vi "solar_voy Pack.vi"(0 "Voyager Refnum in":T1, 1 "CMD":enum8{"CMD", "TLM"}(ring), 2 "Update Last Value? (F)":bool, 5 "TARGET":string, 7 "PACKET (\"\" = Use Variant)":string, 9 "Variant (No HDR)":variant, 11 "error in (no error)":errorcluster, 12 "Suppress Errors? (T)":bool=TRUE, 13 "HDR_GUID":string) -> (4 "Voyager Refnum out":T1, 6 "TCP Data to Send":string, 10 "Packet Index":i32, 15 "error out":errorcluster)   [LabVIEW 2018]
doc: "This packs a variant into a registered TCP packet. The variant should not include the header data. The header items are added automatically."
uses:
  <vilib>/Utility/Data Type/NI_Data Type.lvlib
  solar_voy_ctl Voyager Refnum.ctl
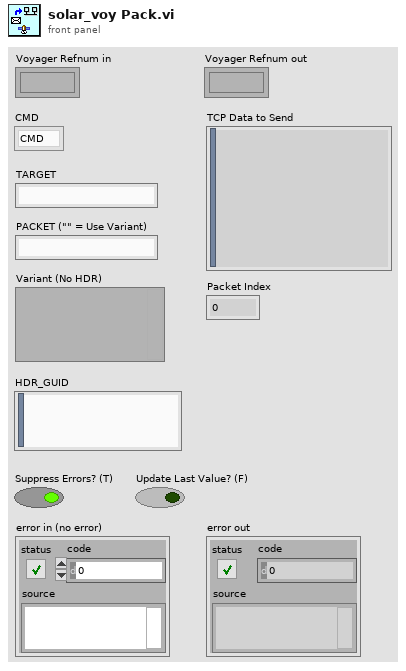
[diagram p1: front panel]
types:
  T1 = typedef "solar_voy_ctl Voyager Refnum.ctl" = refnum<k1>
  T2 = typedef "solar_voy_ctl Voyager.ctl" = cluster{"PACKETS":T3[], "COSMOS_Root":path, "CMD_HDR":T8, "TLM_HDR":T8, "TCPs":T9[], "VoyagerIDOffset":cluster{"VoyagerIDOffset":u16[], "Target Names":string[]}}
  T3 = typedef "solar_voy_def_ctl PACKET.ctl" = cluster{"PACKET_ID":T4, "ENDIAN":enum8{"BIG", "LITTLE"}, "DESC":string, "HZRD":bool, "ITEMS":T5[], "NoExport":bool, "last_time":timestamp, "last_count":u32, "last_data":string}
  T4 = typedef "solar_voy_def_ctl PACKET_ID.ctl" = cluster{"ID":u16, "CMD":enum8{"CMD", "TLM"}, "TARGET":string, "PACKET":string}
  T5 = typedef "solar_voy_def_ctl ITEM.ctl" = cluster{"NAME":string, "OFFSET":i32, "SIZE":i32, "TYPE":T6, "EACH_SIZE":i32, "LVTYPE":T7, "MIN":dbl, "MAX":dbl, "DEFAULT":string, "DESC":string, "ID":bool, "MODIFIERS":variant, "last_value":variant}
  T6 = typedef "solar_voy_def_ctl ITEM TYPE.ctl" = enum8{"BLOCK", "INT", "UINT", "FLOAT", "STRING"}
  T7 = typedef "solar_type Item Type.ctl" = enum16{"NULL", "UNKNOWN", "CLUSTER", "I8", "I16", "I32", "I64", "U8", "U16", "U32", "U64", "U8_ENUM", "U16_ENUM", "U32_ENUM", "SGL", "DBL", "BOOLEAN", "STRING", "PATH", "VISA", "TAG", "TIME", "I8_1D", "I16_1D", "I32_1D", "I64_1D", "U8_1D", "U16_1D", "U32_1D", "U64_1D", "U8_ENUM_1D", "U16_ENUM_1D", "U32_ENUM_1D", "SGL_1D", "DBL_1D", "BOOLEAN_1D", "STRING_1D", "PATH_1D", "VISA_1D", "TAG_1D", "TIME_1D", "I8_2D", "I16_2D", "I32_2D", "I64_2D", "U8_2D", "U16_2D", "U32_2D", "U64_2D", "U8_ENUM_2D", "U16_ENUM_2D", "U32_ENUM_2D", "SGL_2D", "DBL_2D", "BOOLEAN_2D", "STRING_2D", "PATH_2D", "VISA_2D", "TAG_2D", "TIME_2D"}
  T8 = typedef "solar_voy_def_ctl HDR.ctl" = cluster{"ITEMS":T5[], "LENGTH_NAME":string, "LENGTH_VALUE_OFFSET":i32, "ID_NAME":string, "ENDIAN":enum8{"BIG", "LITTLE"}, "GUID_NAME":string, "DEFAULT_TARGET":string, "DEFAULT_PACKET":string, "DEFAULT_ERROR":string}
  T9 = typedef "solar_voy_ctl TCP.ctl" = cluster{"Connected":bool, "Port":u16, "Listener":refnum<k5>, "ServerIP":string, "TCP":refnum<k5>, "Setup":T10, "VIRefnum":refnum<vi>, "TARGETS_CMD":string[], "TARGETS_TLM":string[]}
  T10 = typedef "solar_voy_ctl Port Setup.ctl" = enum8{"SERVER", "CLIENT", "SERVER_CMD", "SERVER_TLM"}
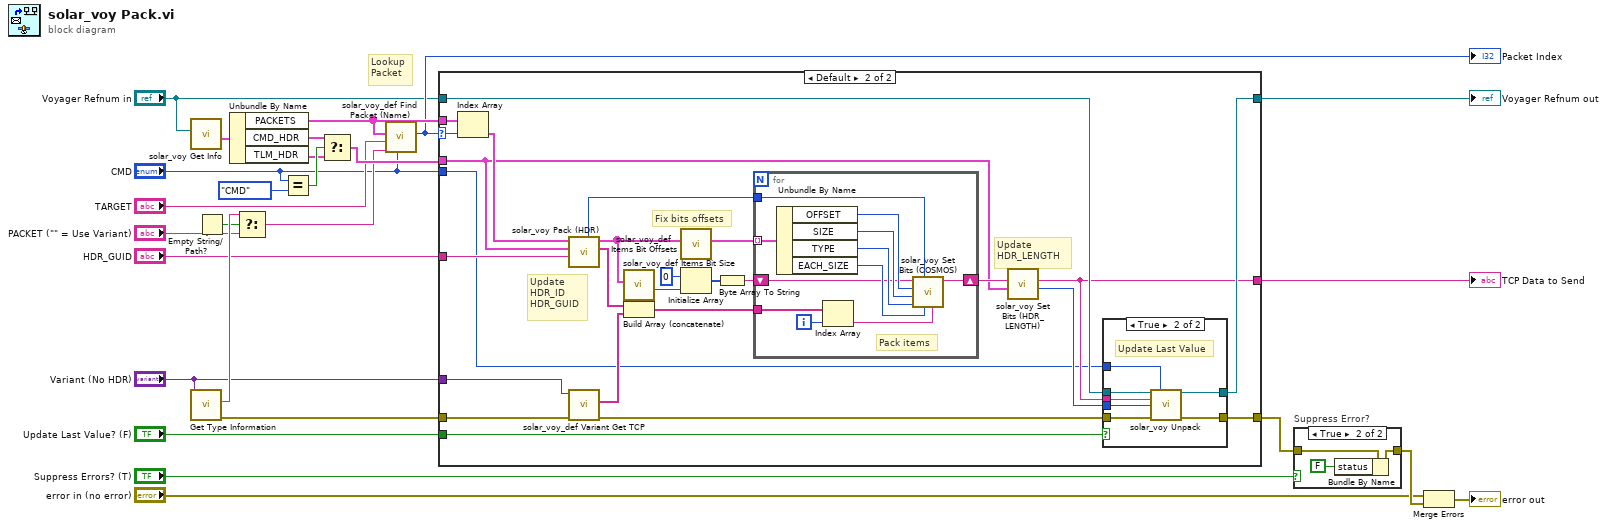
[diagram p0: block diagram]
diagram:
  # "Lookup\nPacket"
  n1 = call "solar_voy Get Info.vi"("Voyager Refnum"="Voyager Refnum in") -> ("Voyager"=w7:T2)  [unwired: 8 in, 2 out]
  n2 = call <vilib>:"Get Type Information.vi"("variant"="Variant (No HDR)") -> ("error out"=w23:errorcluster, "name"=w20:string)  [unwired: 6 in, 3 out]
  n3 = Empty String/Path?(string/path="PACKET (\"\" = Use Variant)") -> (empty?=w18:bool)
  n4 = Unbundle By Name(w7) -> ("PACKETS"=w17:T3[], "CMD_HDR"=w6:T8, "TLM_HDR"=w5:T8)
  n5 = Select(t=w20, s=w18, f="PACKET (\"\" = Use Variant)") -> (s? t:f=w21:string)
  n6 = Equal?(x="CMD", y=enum8{"CMD", "TLM"}."CMD") -> (x = y?=w25:bool)
  n7 = Select(t=w6, s=w25, f=w5) -> (s? t:f=w26:T8)
  n8 = call "solar_voy_def Find Packet (Name).vi"("CMD"="CMD", "PACKET"=w21, "TARGET"="TARGET", "PACKETS"=w17) -> ("Index"=w9:i32)  [unwired: 7 in]
  "Packet Index" <- w9
  n9 = case shown="Default" w9 {
    selector: w9 -> [_ w44]
    tunnel: w26 -> [_ w37]
    tunnel: w23 -> [w28 w49]
    tunnel: [_ w32] -> w22
    tunnel: w17 -> [_ w47]
    tunnel: [w28 w35] -> w13
    tunnel: "HDR_GUID" -> [_ w45]
    tunnel: "Variant (No HDR)" -> [_ w43]
    tunnel: "Voyager Refnum in" -> [w27 w34]
    tunnel: [w27 w33] -> w3
    tunnel: "CMD" -> [_ w30]
    tunnel: "Update Last Value? (F)" -> [_ w29]
    frame -1 {
      # "Packet not found"
    }
    frame Default {
      # "Update\nHDR_LENGTH"
      # "Update\nHDR_ID\nHDR_GUID"
      # "Fix bits offsets"
      n10 = Index Array(array=w47, index=w44) -> (element=w48:T3)
      n11 = call "solar_voy Pack (HDR).vi"("HDR_GUID"=w45, "HDR"=w37, "PACKET"=w48) -> ("HDR LabVIEW Flattened Values"=w41:string[], "ITEMS"=w42:T5[], "ENDIAN"=w40:enum8{"BIG", "LITTLE"})  [unwired: 6 in]
      n12 = call "solar_voy_def Variant Get TCP.vi"("error in (no error)"=w49, "Variant"=w43) -> ("error out"=w36:errorcluster, "LabVIEW Flattened Value"=w39:string[])  [unwired: 7 in, 1 out]
      n13 = call "solar_voy_def Items Bit Size.vi"("ITEMS"=w42) -> ("Byte Size"=w50:i32)  [unwired: 9 in, 1 out]
      n14 = Build Array (concatenate)(w41, w39) -> (w54:string[])
      n15 = call "solar_voy_def Items Bit Offsets.vi"("ITEMS in"=w42) -> ("ITEMS with Bit Offsets"=w46:T5[])  [unwired: 9 in, 1 out]
      n16 = Initialize Array(u8 0, w50) -> (w52:u8[])
      n17 = Byte Array To String(unsigned byte array=w52) -> (string=w53:string)
      n18 = for {
        tunnel: w40 -> [w70]
        tunnel: w46 -> [w68] mode=indexing
        tunnel: w54 -> [w67]
        shift-right: [w64] -> w38
        shift-left: w53 -> [w69]
        i -> [w66]
        # "Pack items"
        n19 = Unbundle By Name(w68) -> ("OFFSET"=w74:i32, "SIZE"=w73:i32, "TYPE"=w72:T6, "EACH_SIZE"=w71:i32)
        n20 = Index Array(array=w67, index=w66) -> (element=w65:string)
        n21 = call "solar_voy Set Bits (COSMOS).vi"("LabVIEW Flattened Value"=w65, "Bit Element Size (Array only)"=w71, "ENDIAN"=w70, "COSMOS TYPE"=w72, "Bit Size"=w73, "Bit Offset"=w74, "Padded COSMOS Data in"=w69) -> ("COSMOS Data out"=w64:string)  [unwired: 2 in, 2 out]
      }
      n22 = call "solar_voy Set Bits (HDR_LENGTH).vi"("HDR"=w37, "TCP Data (No HDR_LENGTH)"=w38) -> ("HDR_ID"=w31:u16, "TCP Data out"=w32:string)  [unwired: 8 in]
      n23 = case shown="True" w29 {
        tunnel: w36 -> [w55 w63]
        tunnel: [w55 w62] -> w35
        tunnel: w34 -> [w56 w61]
        tunnel: [w56 w60] -> w33
        tunnel: w32 -> [_ w59]
        tunnel: w31 -> [_ w58]
        tunnel: w30 -> [_ w57]
        frame False {
        }
        frame True {
          # "Update Last Value"
          n24 = call "solar_voy Unpack.vi"("Voyager Refnum in"=w61, "CMD"=w57, "TCP Data"=w59, "ID"=w58, "error in (no error)"=w63) -> ("Voyager Refnum out"=w60:T1, "error out"=w62:errorcluster)  [unwired: 4 in, 5 out]
        }
      }
    }
  }
  "TCP Data to Send" <- w22
  "Voyager Refnum out" <- w3
  n25 = case "Suppress Error?" shown="True" "Suppress Errors? (T)" {
    tunnel: w13 -> [w75 w78]
    tunnel: [w75 w77] -> w14
    frame False {
    }
    frame True {
      n26 = Bundle By Name(cluster=w78, "status"=FALSE) -> (w77:errorcluster)
    }
  }
  n27 = Merge Errors("error in (no error)", w14) -> (→"error out":errorcluster)
